vi "Get ctrl Secondary Button.vi"(3 "Controls":T1(array[ring])) -> (0 "Array":bool[](array[boolean]))   [LabVIEW 2014]
uses:
  TypeDefs/SRE Enum.ctl
  Support Code/Robot Global Data.vi
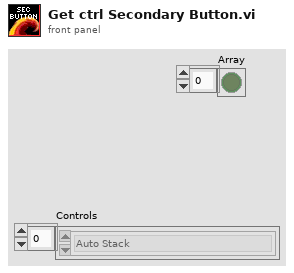
[diagram p1: front panel]
types:
  T1 = enum16{"Auto Stack", "Claw up", "Enable Manuel Elevator", "EM Claw", "Open Claw", "Reset State Machines", "Claw Noodle", "Disable auto stack"}[]
  T2 = typedef "SRE Enum.ctl" = enum16{"Start", "Run", "End"}
  T3 = enum16{"A", "B", "X", "Y", "Left bumper", "Right bumper", "Back", "Start", "Left Joystick down", "Right Joystick down"}[]
  T4 = enum16{"A", "B", "X", "Y", "Left bumper", "Right bumper", "Back", "Start", "Left Joystick down", "Right Joystick down"}
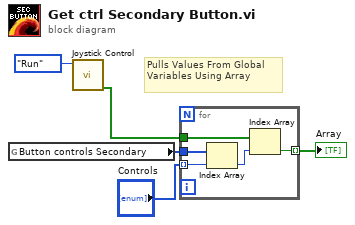
[diagram p0: block diagram]
diagram:
  # "Pulls Values From Global Variables Using Array"
  n1 = global read "Robot Global Data.vi" "Button controls Secondary"() -> (w3:T3)
  n2 = call "Joystick Control.vi"("Enum"=SRE_Enum."Run") -> ("Buttons Output Secondary"=w1:bool[])  [unwired: 3 in, 5 out]
  n3 = for {
    tunnel: "Controls" -> [w10] mode=indexing
    tunnel: [w9] -> w2 mode=indexing
    tunnel: w1 -> [w8]
    tunnel: w3 -> [w6]
    n4 = Index Array(array=w6, index=w10) -> (element=w7:T4)
    n5 = Index Array(array=w8, index=w7) -> (element=w9:bool)
  }
  "Array" <- w2
